vi "PowerTen.vi"() -> ()   [LabVIEW 2011]
panel:
  out "V Mon Scaled (V)":dbl(knob) scale=0.0..40.0
  out "V Mon (V)":dbl(knob) scale=0.0..10.0
  in  "V Mon":i16
  in  "Stop Button":bool
  out "OpenWire":bool
  out "InHold":bool
  out "Fault":bool
  out "Readback (V)":dbl(knob) scale=-10.0..10.0
  out "Output":i16
  in  "Readback":i16
  in  "Output":dbl(knob) min=-10.25 max=10.25 step=0.1 scale=0.0..10.0
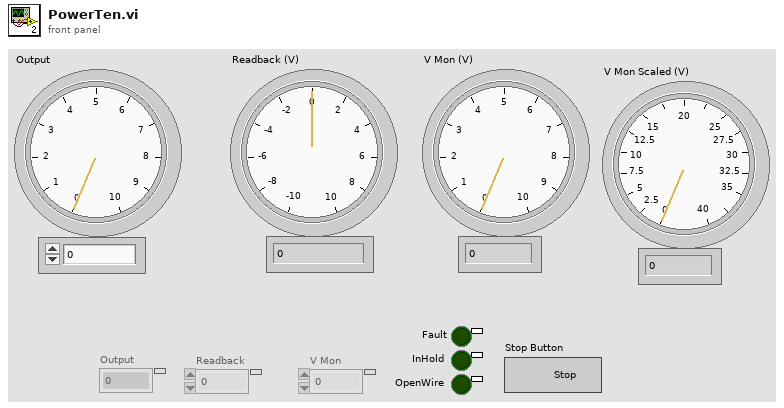
[diagram p1: front panel]
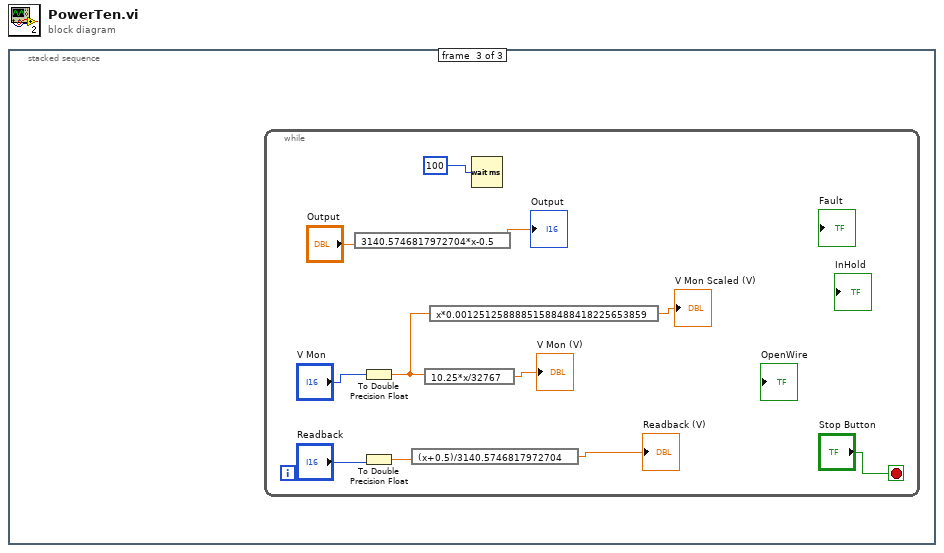
[diagram p0: block diagram]
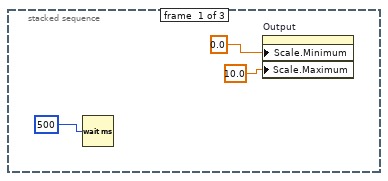
[diagram p2: hidden frame]
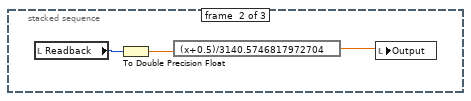
[diagram p3: hidden frame]
diagram:
  n1 = stacked-sequence {
    frame #0 {
      n2 = Wait (ms)(milliseconds to wait=u32 500) -> ()  [unwired: 1 out]
      n3 = property on="Output" class="Knob (strict)"("Scale.Minimum"=0.0, "Scale.Maximum"=10.0) -> ()  [unwired: 2 in, 2 out]
    }
    frame #1 {
      n4 = local read "Readback"() -> (w6:i16)
      n5 = To Double Precision Float(number=w6) -> (double precision float=w5:dbl)
      n6 = expression code="(x+0.5)/3140.5746817972704"(w5) -> (w4:dbl)
      n7 = local write "Output"(w4) -> ()
    }
    frame #2 {
      n8 = while {
        stop <- "Stop Button" stop-if-true
        n9 = expression code="3140.5746817972704*x-0.5"("Output") -> (→"Output":dbl)
        n10 = To Double Precision Float(number="V Mon") -> (double precision float=w7:dbl)
        n11 = To Double Precision Float(number="Readback") -> (double precision float=w13:dbl)
        n12 = expression code="(x+0.5)/3140.5746817972704"(w13) -> (→"Readback (V)":dbl)
        n13 = expression code="10.25*x/32767"(w7) -> (→"V Mon (V)":dbl)
        n14 = expression code="x*0.00125125888851588488418225653859"(w7) -> (→"V Mon Scaled (V)":dbl)
        n15 = Wait (ms)(milliseconds to wait=u32 100) -> ()  [unwired: 1 out]
      }
    }
  }
